vi "GREENHEAVEN3.vi"() -> ()   [LabVIEW 2025]
uses:
  <vilib>/Instr/_visa.llb/VISA Configure Serial Port (Instr).vi
panel:
  in  "HUMIDITY":bool
  in  "SOIL":bool
  in  "BUZZER":bool
  in  "TDS":bool
  in  "WATER":bool
  out "TDS":dbl(slide) scale=0.0..100.0
  out "TDS \nINDICATOR":bool
  out "ROOM TEMPMERETURE \nINDICATOR (BUZZER)":bool
  out "WATER TEMPERETURE \nINDICATOR":bool
  out "HUMIDITY INDICATOR":bool
  out "SOIL MOISTURE \nINDICATOR":bool
  in  "TDS Range":dbl(slide) scale=0.0..100.0
  in  "Water Tempereture Range":dbl(slide) scale=0.0..100.0
  in  "Soil Moisture Range":dbl(slide) scale=0.0..100.0
  in  "Room Tempereture Range":dbl(slide) scale=0.0..100.0
  out "Room \nTempereture":dbl(slide) scale=0.0..100.0 scale format="%#.4g"
  out "Humidity":dbl(slide) scale=0.0..100.0 scale format="%#_4g"
  out "Soil Moisture":dbl(slide) scale=0.0..100.0
  out "Water \nTempereture":dbl(slide) scale=0.0..100.0 scale format="%#_4g"
  in  "PORT":refnum<visa-resource-name>
  in  "?":bool
  # "MANNUAL BUTTONS"
  # "GREEN HEAVEN (SMART HOME GARDEN SYSTEM)"
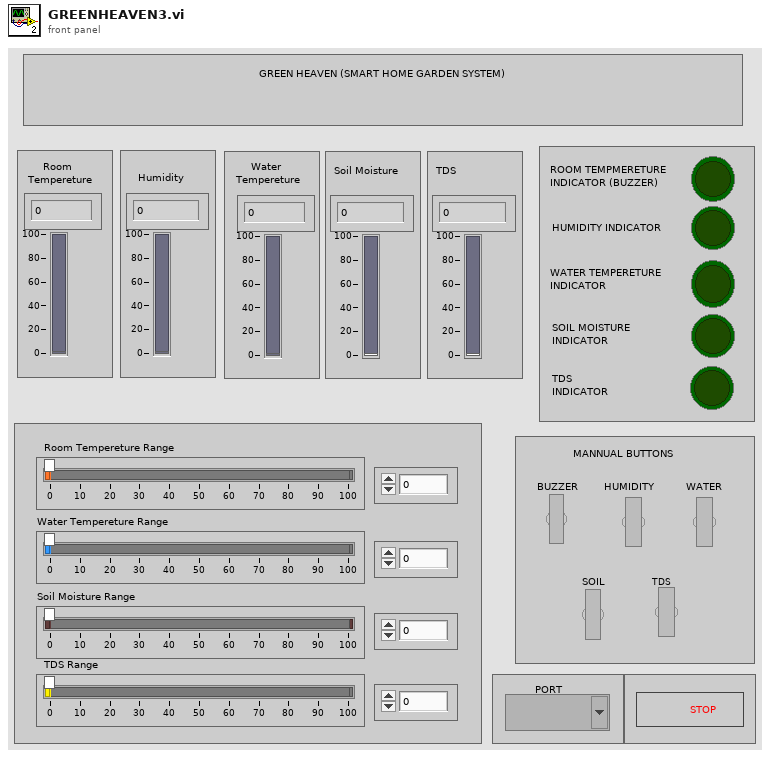
[diagram p1: front panel]
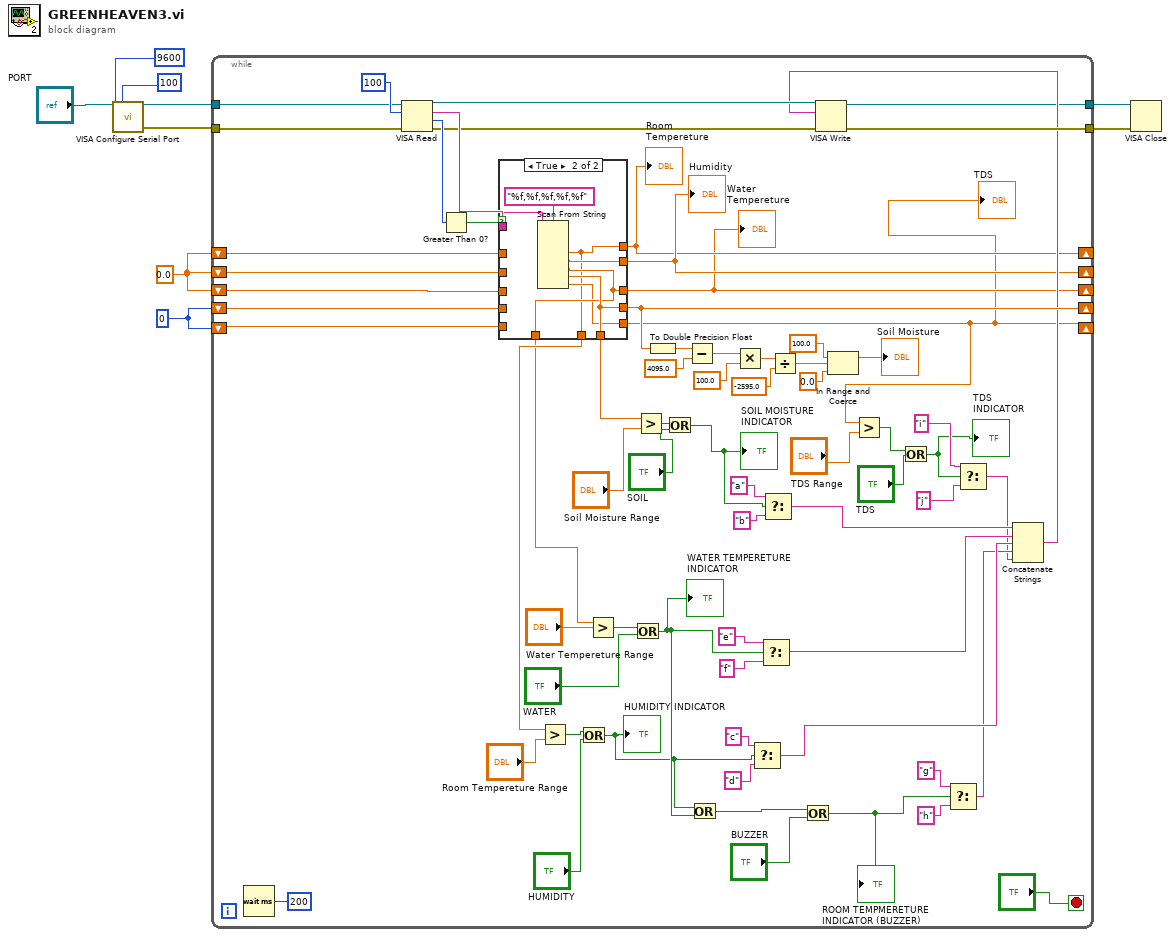
[diagram p0: block diagram]
diagram:
  w1 = 0
  w3 = 0.0
  n1 = call-poly "VISA Configure Serial Port"("VISA resource name"="PORT", "timeout (10sec)"=u32 100, "baud rate (9600)"=u32 9600) -> ("VISA resource name out"=w9:refnum<visa-resource-name>, "error out"=w8:errorcluster)  [unwired: 11 in]
  n2 = while {
    tunnel: w9 -> [w76]
    tunnel: w8 -> [w75]
    tunnel: [w78] -> w7
    shift-right: [w29] -> _
    shift-left: w3 -> [w67]
    shift-right: [w30] -> _
    shift-left: w3 -> [w69]
    shift-right: [w15] -> _
    shift-left: w3 -> [w68]
    shift-right: [w56] -> _
    shift-left: w1 -> [w66]
    tunnel: [w26] -> w2
    shift-right: [w13] -> _
    shift-left: w1 -> [w23]
    stop <- "?" stop-if-true
    n3 = Wait (ms)(milliseconds to wait=u32 200) -> ()  [unwired: 1 out]
    n4 = VISA Read(VISA resource name=w76, byte count=u32 100, error in (no error)=w75) -> (VISA resource name out=w73:refnum<visa-resource-name>, read buffer=w74:string, return count=w71:u32, error out=w27:errorcluster)
    n5 = Greater Than 0?(x=w71) -> (x > 0?=w70:bool)
    n6 = case shown="True" w70 {
      tunnel: w74 -> [_ w91]
      tunnel: w67 -> [w84 _]
      tunnel: w69 -> [w82 _]
      tunnel: w68 -> [w81 _]
      tunnel: w66 -> [w83 _]
      tunnel: [w84 w85] -> w29
      tunnel: [w82 w88] -> w30
      tunnel: [w81 w87] -> w15
      tunnel: [w83 w89] -> w56
      tunnel: [w83 w89] -> w55
      tunnel: [w82 w85] -> w47
      tunnel: [w81 w87] -> w44
      tunnel: [w80 w86] -> w13
      tunnel: w23 -> [w80 _]
      frame False {
      }
      frame True {
        n7 = Scan From String(format string="%f,%f,%f,%f,%f", input string=w91) -> (output 1=w85:dbl, output 2=w88:dbl, output 3=w87:dbl, output 4=w89:dbl, output 5=w86:dbl)  [unwired: 7 in, 3 out]
      }
    }
    "Water \nTempereture" <- w15
    "Room \nTempereture" <- w29
    "Humidity" <- w30
    "TDS" <- w13
    n8 = Greater?(x=w47, y="Room Tempereture Range") -> (0:w11:bool)
    n9 = Or(x=w11, y="HUMIDITY") -> (x .or. y?=w12:bool)
    "HUMIDITY INDICATOR" <- w12
    n10 = Greater?(x=w44, y="Water Tempereture Range") -> (0:w25:bool)
    n11 = Or(x=w25, y="WATER") -> (x .or. y?=w14:bool)
    "WATER TEMPERETURE \nINDICATOR" <- w14
    n12 = Greater?(x=w55, y="Soil Moisture Range") -> (0:w53:bool)
    n13 = To Double Precision Float(number=w56) -> (double precision float=w65:dbl)
    n14 = Or(x=w53, y="SOIL") -> (x .or. y?=w51:bool)
    "SOIL MOISTURE \nINDICATOR" <- w51
    n15 = Subtract(x=w65, y=4095.0) -> (x-y=w63:dbl)
    n16 = Or(x=w12, y=w14) -> (x .or. y?=w40:bool)
    n17 = Multiply(x=w63, y=100.0) -> (x*y=w61:dbl)
    n18 = Select(t="c", s=w12, f="d") -> (s? t:f=w33:string)
    n19 = Select(t="e", s=w14, f="f") -> (s? t:f=w34:string)
    n20 = Select(t="a", s=w51, f="b") -> (s? t:f=w35:string)
    n21 = Divide(x=w61, y=-2595.0) -> (x/y=w59:dbl)
    n22 = Or(x=w40, y="BUZZER") -> (x .or. y?=w38:bool)
    "ROOM TEMPMERETURE \nINDICATOR (BUZZER)" <- w38
    n23 = In Range and Coerce(upper limit=100.0, x=w59, lower limit=0.0) -> (coerced(x)=→"Soil Moisture":dbl)  [unwired: 1 out]
    n24 = Greater?(x=w13, y="TDS Range") -> (0:w18:bool)
    n25 = Or(x=w18, y="TDS") -> (x .or. y?=w17:bool)
    "TDS \nINDICATOR" <- w17
    n26 = Select(t="g", s=w38, f="h") -> (s? t:f=w32:string)
    n27 = Select(t="i", s=w17, f="j") -> (s? t:f=w22:string)
    n28 = Concatenate Strings(w35, w34, w33, w32, w22) -> (w31:string)
    n29 = VISA Write(VISA resource name=w73, write buffer=w31, error in (no error)=w27) -> (VISA resource name out=w26:refnum<visa-resource-name>, error out=w78:errorcluster)  [unwired: 1 out]
  }
  n30 = VISA Close(VISA resource name=w2, error in (no error)=w7) -> ()  [unwired: 1 out]
